vi "GetType&ID.vi"(8 "Error In":errorcluster, 10 "Plugin reference out":refnum<class "ModuleAdmin.lvclass">, 11 "AcPwrBase in":refnum<class "AcPwrBase.lvclass">) -> (0 "Error Out":errorcluster, 1 "Cluster":T1, 2 "reference out":refnum<class "ModuleAdmin.lvclass">, 3 "AcPwrBase out":refnum<class "AcPwrBase.lvclass">)   [LabVIEW 2018, in "AcPwrPlugins.lvlib" / "AcPwrBase.lvclass"]
uses:
  AcPwrBase.lvclass
  <userlib>/NIST/ModuleAdminLib/ModuleAdmin/ModuleAdmin.lvclass
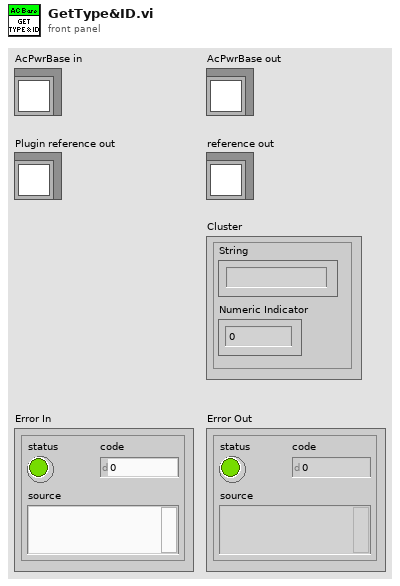
[diagram p1: front panel]
types:
  T1 = cluster{"String":string, "Numeric Indicator":i32}
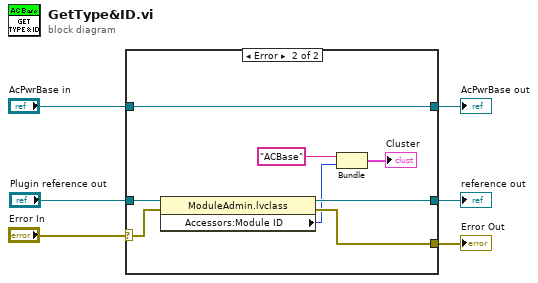
[diagram p0: block diagram]
diagram:
  n1 = case shown="Error" "Error In" {
    selector: "Error In" -> [w9 w14]
    tunnel: "AcPwrBase in" -> [w8 w17]
    tunnel: [w9 w13] -> w4
    tunnel: [w8 w17] -> w3
    tunnel: "Plugin reference out" -> [w7 w16]
    tunnel: [w7 w15] -> w1
    frame No Error {
    }
    frame Error {
      n2 = property class="ModuleAdmin.lvclass"(reference=w16, error in=w14) -> (reference out=w15:refnum<class "ModuleAdmin.lvclass">, error out=w13:errorcluster, "Accessors:Module ID"=w11:i32)
      n3 = Bundle("ACBase", "Accessors:Module ID"=w11) -> (→"Cluster":cluster{string, "Accessors:Module ID":i32})  [unwired: 1 in]
    }
  }
  "AcPwrBase out" <- w3
  "Error Out" <- w4
  "reference out" <- w1
